vi "createdatafolder.vi"(0 "timestamp in":timestamp) -> (1 "current data path":path, 2 "timestamp out":timestamp)   [LabVIEW 2015]
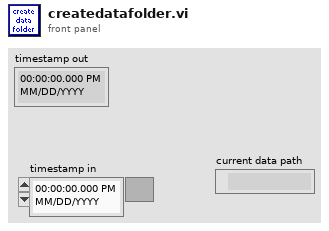
[diagram p1: front panel]
types:
  T1 = cluster{"StageS":i32, "StageL":i32, "currmeas data dir":path, "image OD":u16, "contour OD":u16, "point OD":u16, "AOlines":tag[], "AIlines":tag[], "CI lines":tag[], "DO lines":tag[], "AO names":string[], "CI names":string[], "AI names":string[], "DO names":string[], "CIextensions":string[], "AIextensions":string[], "Voltage to Ygalvo":i32, "Voltage to Xgalvo":i32, "Voltage to patch":i32, "640 shutter":i32, "2P shutter":i32, "LT timestamp":u32, "Vp":i32, "Ip":i32, "camera trigger":i32, "master data dir":path, "voltage to Zpos":i32, "Vto2P":i32, "640 AO":i32, "488 AO":i32, "532 AO":i32, "640TTL":u32, "488TTL":u32, "532TTL":u32, "Device 1 sampleclock out":tag, "Device 1 Starttrigger out":tag, "Device 2 sampleclock in":tag, "Device 2 StartTrigger in ":tag, "2PODTTL":u32, "488 shutter":u32, "LCVR red":u32, "LCVR blue":u32}
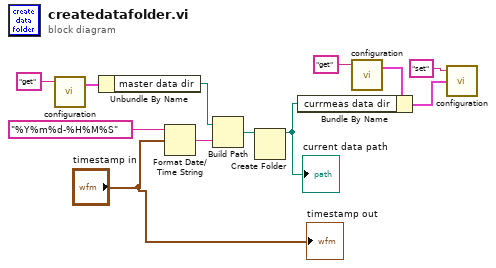
[diagram p0: block diagram]
diagram:
  n1 = call "configuration.vi"("command"="get") -> ("config out"=w5:T1)  [unwired: 2 in, 1 out]
  n2 = Unbundle By Name(w5) -> ("master data dir"=w4:path)
  n3 = Format Date/Time String(time format string (%c)="%Y%m%d-%H%M%S", seconds (now)="timestamp in") -> (date/time string=w8:string)  [unwired: 1 in]
  n4 = Build Path(base path=w4, name or relative path=w8) -> (appended path=w3:path)
  n5 = Create Folder(path (use dialog)=w3) -> (created path=w2:path)  [unwired: 2 in, 2 out]
  "current data path" <- w2
  n6 = call "configuration.vi"("command"="get") -> ("config out"=w12:T1)  [unwired: 2 in, 1 out]
  n7 = Bundle By Name(cluster=w12, "currmeas data dir"=w2) -> (w11:T1)
  n8 = call "configuration.vi"("config in"=w11, "command"="set") -> ()  [unwired: 1 in, 2 out]
  "timestamp out" <- "timestamp in"
